vi "Degrees to the right target.vi"(1 "Distance to Target (ft)":dbl, 2 "Distance to Wall (ft)":dbl) -> (0 "Degrees to Right Target":dbl)   [LabVIEW 2013]
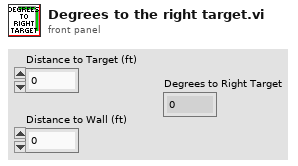
[diagram p1: front panel]
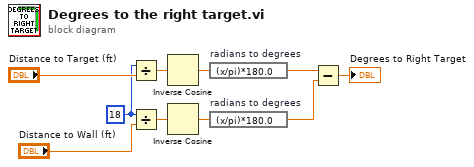
[diagram p0: block diagram]
diagram:
  w8 = 18
  n1 = Divide(x=w8, y="Distance to Target (ft)") -> (x/y=w7:dbl)
  n2 = Divide(x=w8, y="Distance to Wall (ft)") -> (x/y=w6:dbl)
  n3 = Inverse Cosine(1:w7) -> (0:w4:dbl)
  n4 = Inverse Cosine(1:w6) -> (0:w5:dbl)
  n5 = expression code="(x/pi)*180.0" "radians to degrees"(w4) -> (w3:dbl)
  n6 = expression code="(x/pi)*180.0" "radians to degrees"(w5) -> (w2:dbl)
  n7 = Subtract(x=w3, y=w2) -> (x-y=→"Degrees to Right Target":dbl)
